vi "ErrorCheckHWI.vi"(8 "error in (no error)":errorcluster, 11 "Novatech in":refnum<class "Novatech.lvclass">) -> (0 "error out":errorcluster, 3 "Novatech out":refnum<class "Novatech.lvclass">)   [LabVIEW 2013, in "Novatech.lvclass"]
uses:
  Novatech.lvclass
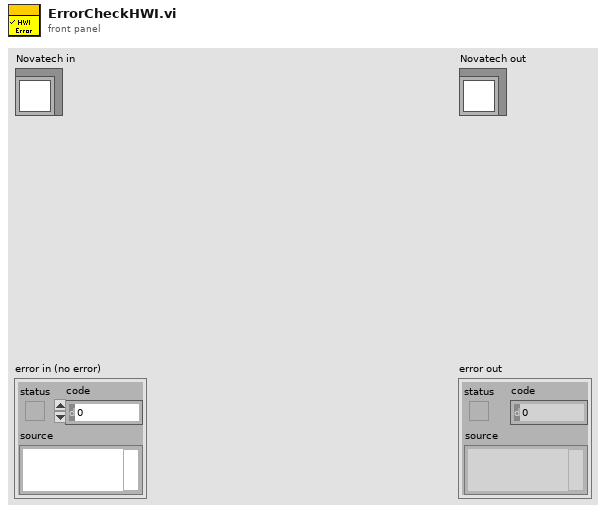
[diagram p1: front panel]
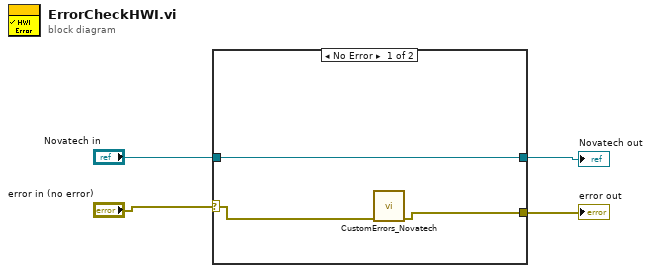
[diagram p0: block diagram]
diagram:
  n1 = case shown="No Error" "error in (no error)" {
    selector: "error in (no error)" -> [w7 w8]
    tunnel: [w6 w8] -> w3
    tunnel: [w5 w9] -> w2
    tunnel: "Novatech in" -> [w5 w9]
    frame No Error {
      n2 = call "CustomErrors_Novatech.vi"("error in (no error)"=w7) -> ("error out"=w6:errorcluster)  [unwired: 10 in]
    }
    frame Error {
    }
  }
  "error out" <- w3
  "Novatech out" <- w2
